vi "Write Value.vi"(8 "error in":errorcluster, 10 "val":u8, 11 "PowerSupply MSG in":refnum<class "PowerSupply MSG.lvclass">) -> (0 "error out":errorcluster, 3 "PowerSupply MSG out":refnum<class "PowerSupply MSG.lvclass">)   [LabVIEW 2014, in "Controller.lvlib" / "PowerSupply MSG.lvclass"]
uses:
  PowerSupply MSG.lvclass
  PowerSupply MSG.lvclass/PowerSupply MSG.ctl
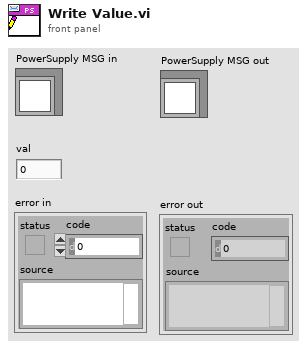
[diagram p1: front panel]
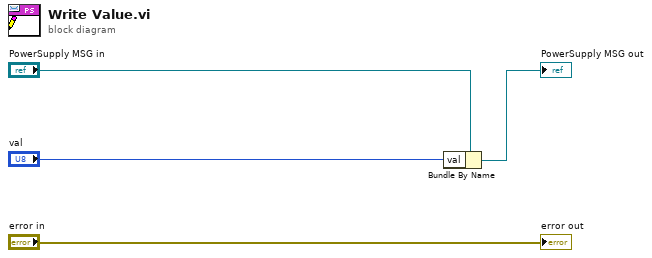
[diagram p0: block diagram]
diagram:
  n1 = Bundle By Name(cluster="PowerSupply MSG in", "val"="val") -> (→"PowerSupply MSG out":refnum<class "PowerSupply MSG.lvclass">)
  "error out" <- "error in"
